vi "Check for GFG variables in Settings array.vi"(8 "error in (no error)":errorcluster, 10 "GFG variables to search":string[](array[string]), 11 "Settings ArrayIN":T1[](array[typedef])) -> (0 "error out":errorcluster, 1 "GFG ariables not found":string[](array[string]), 2 "GFG variant values (those found)":variant[](array[variant]), 3 "GFG variables found":string[](array[string]), 4 "Error Message (list of variables not found)":string, 5 "Any Not Found?":bool)   [LabVIEW 2012]
doc: "SciScan 1.2 160622\nThis VI checks a settings array if another every GFG variable specified in another input (string) array is present.\nThe VI outputs array of found GFG Variables, their corresponding Variant values, array of variables not found, and an error message (if any) specifying the variables that were not found"
uses:
  MacroGUI Module/Custom Controls and Typedefs/GFG Variable for IO.ctl
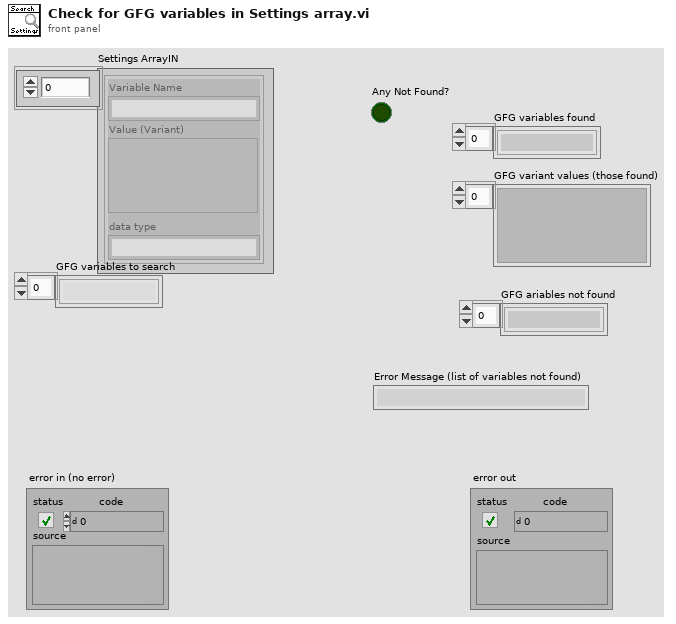
[diagram p1: front panel]
types:
  T1 = typedef "GFG Variable for IO.ctl" = cluster{"Variable Name":string, "Value (Variant)":variant, "data type":string}
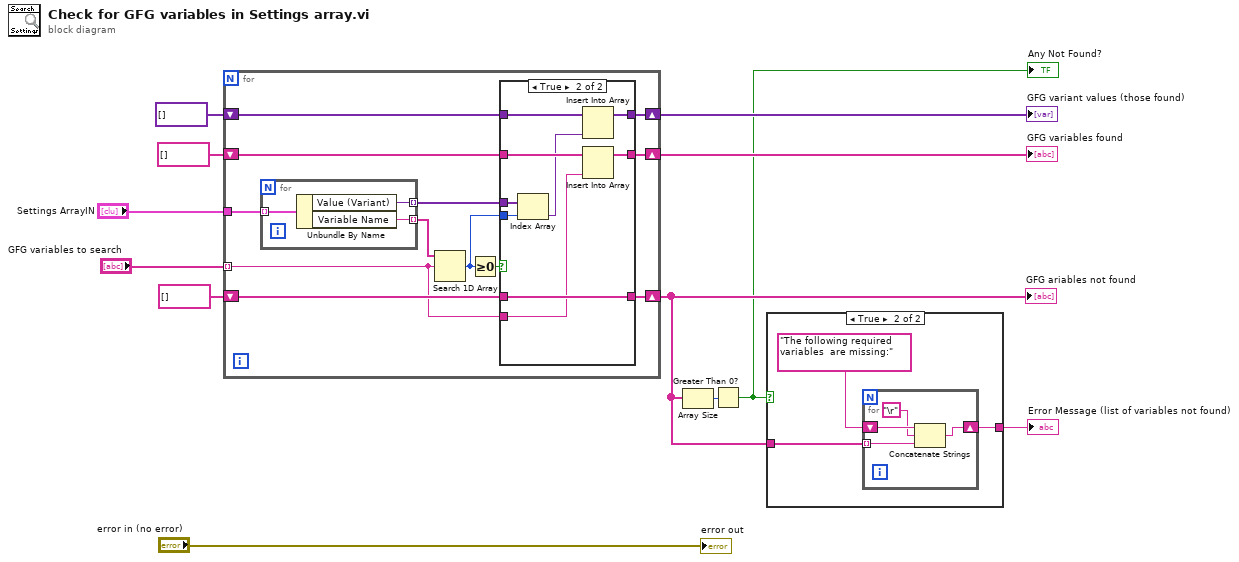
[diagram p0: block diagram]
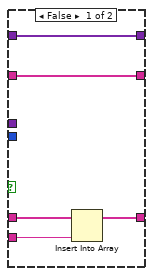
[diagram p3: hidden frame]
diagram:
  n1 = for {
    tunnel: "Settings ArrayIN" -> [w24]
    tunnel: "GFG variables to search" -> [w20] mode=indexing
    shift-right: [w19] -> w3
    shift-left: string[] [] -> [w21]
    shift-right: [w15] -> w7
    shift-left: variant[] [] -> [w18]
    shift-right: [w16] -> w6
    shift-left: string[] [] -> [w17]
    n2 = for {
      tunnel: w24 -> [w41] mode=indexing
      tunnel: [w40] -> w23 mode=indexing
      tunnel: [w39] -> w14 mode=indexing
      n3 = Unbundle By Name(w41) -> ("Value (Variant)"=w39:variant, "Variable Name"=w40:string)
    }
    n4 = Search 1D Array(1D array=w23, element=w20) -> (index of element=w13:i32)  [unwired: 1 in]
    n5 = Greater Or Equal To 0?(x=w13) -> (x >= 0?=w22:bool)
    n6 = case shown="True" w22 {
      tunnel: w21 -> [w29 w34]
      tunnel: w20 -> [w28 w33]
      tunnel: [w27 w34] -> w19
      tunnel: w18 -> [w25 w38]
      tunnel: w17 -> [w26 w37]
      tunnel: [w26 w36] -> w16
      tunnel: [w25 w35] -> w15
      tunnel: w14 -> [_ w32]
      tunnel: w13 -> [_ w31]
      frame False {
        n7 = Insert Into Array(array=w29, new element=w28) -> (w27:string[])  [unwired: 1 in]
      }
      frame True {
        n8 = Index Array(array=w32, index=w31) -> (element=w30:variant)
        n9 = Insert Into Array(array=w38, new element=w30) -> (w35:variant[])  [unwired: 1 in]
        n10 = Insert Into Array(array=w37, new element=w33) -> (w36:string[])  [unwired: 1 in]
      }
    }
  }
  "GFG variant values (those found)" <- w7
  "GFG variables found" <- w6
  "GFG ariables not found" <- w3
  n11 = Array Size(array=w3) -> (size(s)=w4:i32)
  n12 = Greater Than 0?(x=w4) -> (x > 0?=w1:bool)
  "Any Not Found?" <- w1
  n13 = case shown="True" w1 {
    tunnel: w3 -> [_ w43]
    tunnel: [_ w42] -> w2
    frame False {
    }
    frame True {
      n14 = for {
        shift-right: [w45] -> w42
        shift-left: "The following required variables  are missing:" ("Variable Name in") -> [w48]
        tunnel: w43 -> [w46] mode=indexing
        n15 = Concatenate Strings(w48, "\r", w46) -> (w45:string)
      }
    }
  }
  "Error Message (list of variables not found)" <- w2
  "error out" <- "error in (no error)"
